vi "Refresh Warnings.vi"(8 "error in":errorcluster, 9 "Source":string, 10 "Code":string, 11 "Fault Handler in":refnum<class "Fault Handler.lvclass">) -> (0 "error out":errorcluster, 3 "Fault Handler out":refnum<class "Fault Handler.lvclass">)   [LabVIEW 2019, in "Fault Handler.lvlib" / "Fault Handler.lvclass"]
doc: "Called when warning data is provided. \nThis routine checks the active warning data to confirm if the warning is already active: \n\n<b>Warning Already Active</b>\nThe routine skips all additional steps and calls <b>Refresh Display</b>\n\n<b>Warning Not Active</b>\nThe warning is added to the active warning list and constructs a warning log record\nThe log record is written to the warning log output file and appended to the warning history indicator\nThe routine calls <b>Refresh Display</b>"
uses:
  Project/Fault Handler.lvclass
  Project/Fault Handler.lvclass/Fault Handler.ctl
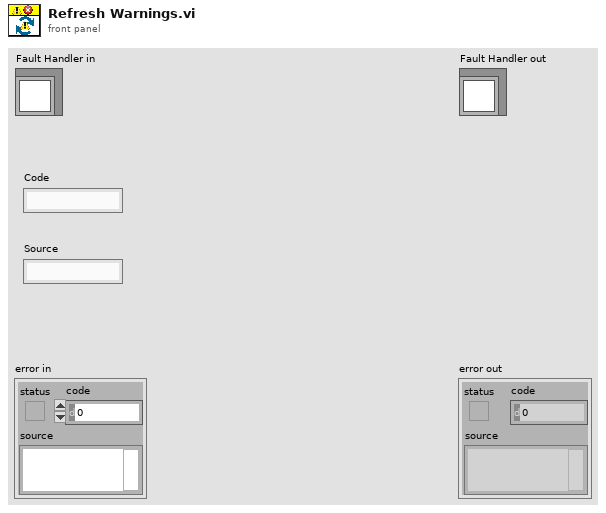
[diagram p1: front panel]
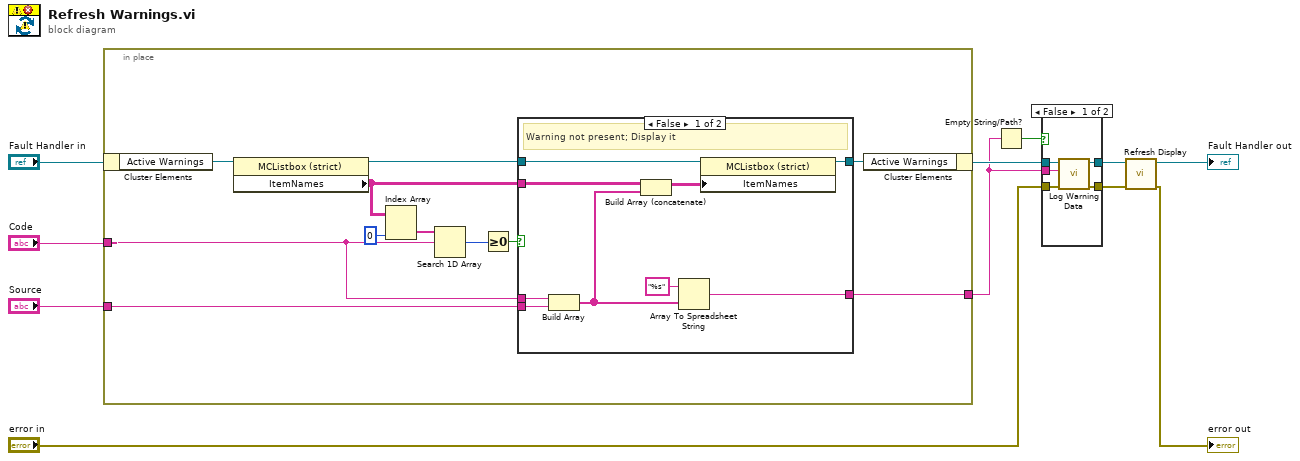
[diagram p0: block diagram]
diagram:
  n1 = in-place {
    in-place-border: "Code" -> [w14]
    in-place-border: "Source" -> [w13]
    in-place-border: [w12] -> w2
    n2 = in-place-cluster #1("Fault Handler in") -> ("Active Warnings"=w22:refnum<vi>)
    n3 = property class="MCListbox (strict)"(reference=w22) -> (reference out=w17:refnum<vi>, "ItemNames"=w16:string[][])  [unwired: 1 in, 1 out]
    n4 = Index Array(array=w16, index (col)=0) -> (element=w20:string[])  [unwired: 1 in]
    n5 = Search 1D Array(1D array=w20, element=w14) -> (index of element=w19:i32)  [unwired: 1 in]
    n6 = Greater Or Equal To 0?(x=w19) -> (x >= 0?=w18:bool)
    n7 = case shown="False" w18 {
      tunnel: w17 -> [w31 w32]
      tunnel: [w30 w32] -> w15
      tunnel: w14 -> [w29 _]
      tunnel: w13 -> [w28 _]
      tunnel: w16 -> [w27 _]
      tunnel: [w24 _] -> w12
      frame False {
        # "Warning not present; Display it"
        n8 = Build Array(w29, w28) -> (w25:string[])
        n9 = Build Array (concatenate)(w27, w25) -> (w26:string[][])
        n10 = Array To Spreadsheet String(array=w25, 3:"%s" ("format string")) -> (spreadsheet string=w24:string)  [unwired: 1 in]
        n11 = property class="MCListbox (strict)"(reference=w31, "ItemNames"=w26) -> (reference out=w30:refnum<vi>)  [unwired: 1 in, 1 out]
      }
      frame True {
        # "Warning Already Present; do not duplicate"
      }
    }
    n12 = in-place-cluster #1("Active Warnings"=w15) -> (w6:refnum<class "Fault Handler.lvclass">)
  }
  n13 = Empty String/Path?(string/path=w2) -> (empty?=w1:bool)
  n14 = case shown="False" w1 {
    tunnel: w6 -> [w37 w39]
    tunnel: [w36 w39] -> w5
    tunnel: [w35 w38] -> w4
    tunnel: "error in" -> [w34 w38]
    tunnel: w2 -> [w33 _]
    frame False {
      n15 = call "Log Warning Data.vi"("error in"=w34, "Warning Data"=w33, "Fault Handler in"=w37) -> ("error out"=w35:errorcluster, "Fault Handler out"=w36:refnum<class "Fault Handler.lvclass">)  [unwired: 7 in]
    }
    frame True {
    }
  }
  n16 = call "Refresh Display.vi"("error in"=w4, "Fault Handler in"=w5) -> ("error out"=→"error out":errorcluster, "Fault Handler out"=→"Fault Handler out":refnum<class "Fault Handler.lvclass">)  [unwired: 8 in]
